vi "Init.vi"(7 "Sender":refnum<class "Sender.lvclass">) -> (3 "Destroy Self Msg out":refnum<class "Destroy Self Msg.lvclass">)   [LabVIEW 2025, in "jettl.lvlib" / "Destroy Self Msg.lvlib" / "Destroy Self Msg.lvclass"]
uses:
  Destroy Self Msg.lvclass
  Destroy Self Msg.lvclass/Destroy Self Msg.ctl
  Sender/Sender/Sender.lvclass
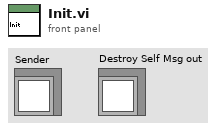
[diagram p1: front panel]
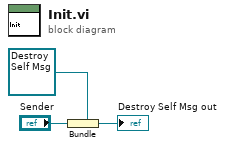
[diagram p0: block diagram]
diagram:
  n1 = Bundle "Bundle"(cluster=refnum<class "Destroy Self Msg.lvclass"> refnum ("Destroy Msg in"), "Sender") -> (→"Destroy Self Msg out":refnum<class "Destroy Self Msg.lvclass">)
